vi "TestRFGVFlag Status.vi"() -> (0 "error out":errorcluster, 2 "Pass":bool)   [LabVIEW 2015]
uses:
  LVClasses/Flags/ColorFlags.ctl
  TypeDef/RoomsActionEnum.ctl
  LVClasses/Flags/Flags.lvclass
panel:
  out "JSON string":string
  out "Data Out 2":string
  out "Data Out":string
  in  "State":bool[](array[boolean])=[FALSE, FALSE, FALSE, FALSE]
  out "Flags Read 1":T1={"Flag State"=[1, 3, 5, 7]}
  out "Flags Write":T1={"Flag State"=[1, 3, 5, 7]}
  out "Flags Read 2":T1={"Flag State"=[1, 3, 5, 7]}
  in  "FGV Room":i32=102
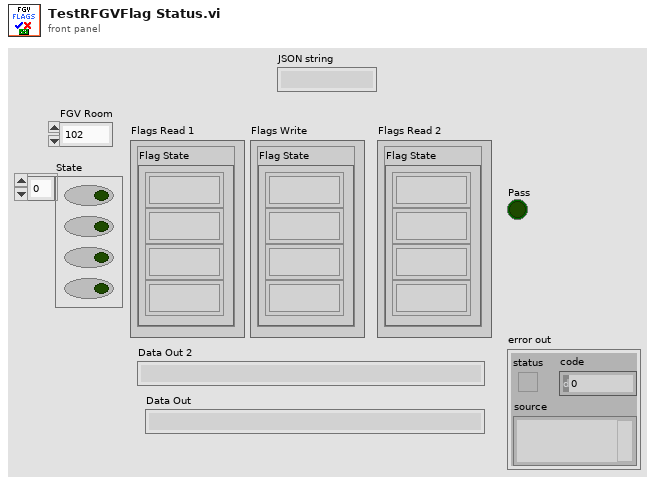
[diagram p1: front panel]
types:
  T1 = typedef "Flags.lvclass/ColorFlags.ctl" = cluster{"Flag State":u8[]}
  T2 = typedef "RoomsActionEnum.ctl" = enum16{"Init", "Add Room", "Remove Room", "Read Room", "Read Flag", "Read Flag State", "Write Flag State", "Read Flag Color", "Write Flag Color", "Read Bed Vacant", "Write Bed Vacant", "Read Personnel", "Add Personnel", "Remove Personnel", "Read Requests", "Add Request", "Remove Request", "Read Beacon ID", "Write Beacon ID", "Write Bed URL", "Read Bed URL", "Read Rooms Numbers", "Write Flag"}
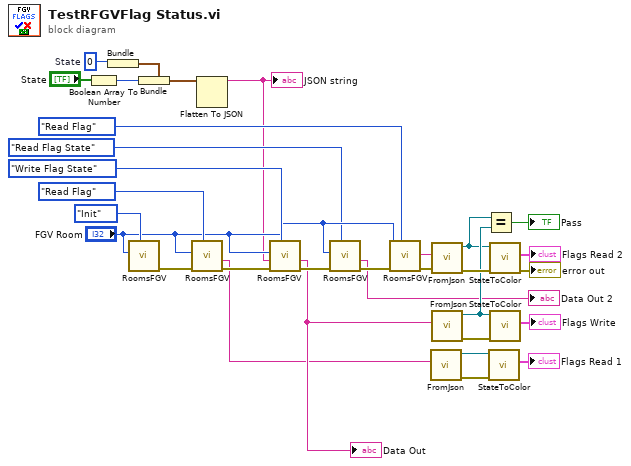
[diagram p0: block diagram]
diagram:
  w4 = u32 0  # State
  n1 = Boolean Array To Number(Boolean array="State") -> (number=w3:u32)
  n2 = Bundle("State"=w4) -> (w2:cluster{"State":u32})  [unwired: 1 in]
  n3 = call "RoomsFGV.vi"("Actions"=RoomsActionEnum."Init", "Room"="FGV Room") -> ("error out"=w31:errorcluster)  [unwired: 8 in, 1 out]
  n4 = Bundle(cluster=w2, "State"=w3) -> (w1:cluster{"State":u32})
  n5 = call "RoomsFGV.vi"("Actions"=RoomsActionEnum."Read Flag", "error in (no error)"=w31, "Room"="FGV Room") -> ("error out"=w30:errorcluster, "Data Out"=w17:string)  [unwired: 7 in]
  n6 = Flatten To JSON(anything=w1) -> (JSON string=w5:string)  [unwired: 2 in, 1 out]
  "JSON string" <- w5
  n7 = call "RoomsFGV.vi"("Actions"=RoomsActionEnum."Write Flag State", "error in (no error)"=w30, "Data In"=w5, "Room"="FGV Room") -> ("error out"=w29:errorcluster, "Data Out"=w18:string)  [unwired: 6 in]
  "Data Out" <- w18
  n8 = call "RoomsFGV.vi"("Actions"=RoomsActionEnum."Read Flag State", "error in (no error)"=w29, "Room"="FGV Room") -> ("error out"=w10:errorcluster, "Data Out"=→"Data Out 2":string)  [unwired: 7 in]
  n9 = call "RoomsFGV.vi"("Actions"=RoomsActionEnum."Read Flag", "error in (no error)"=w10, "Room"="FGV Room") -> ("error out"=w26:errorcluster, "Data Out"=w19:string)  [unwired: 7 in]
  n10 = call "FromJson.vi"("String"=w17) -> ("error out"=w21:errorcluster, "Flags out"=w15:refnum<class "Flags.lvclass">)  [unwired: 9 in]
  n11 = call "FromJson.vi"("error in (no error)"=w26, "String"=w19) -> ("error out"=w25:errorcluster, "Flags out"=w6:refnum<class "Flags.lvclass">)  [unwired: 8 in]
  n12 = call "FromJson.vi"("String"=w18) -> ("error out"=w22:errorcluster, "Flags out"=w16:refnum<class "Flags.lvclass">)  [unwired: 9 in]
  n13 = Equal?(x=w6, y=w16) -> (x = y?=→"Pass":bool)
  n14 = call "StateToColor.vi"("error in (no error)"=w21, "Flags in"=w15) -> ("RoomNumFlags"=→"Flags Read 1":T1)  [unwired: 7 in, 2 out]
  n15 = call "StateToColor.vi"("error in (no error)"=w25, "Flags in"=w6) -> ("error out"=→"error out":errorcluster, "RoomNumFlags"=→"Flags Read 2":T1)  [unwired: 7 in, 1 out]
  n16 = call "StateToColor.vi"("error in (no error)"=w22, "Flags in"=w16) -> ("RoomNumFlags"=→"Flags Write":T1)  [unwired: 7 in, 2 out]
